vi "labpower.vi"() -> ()   [LabVIEW 2019]
panel:
  in  "Numeric":dbl
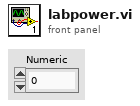
[diagram p1: front panel]
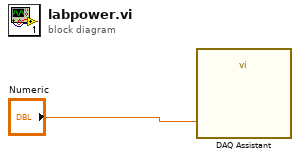
[diagram p0: block diagram]
diagram:
  n1 = call "DAQ Assistant"("data"="Numeric") -> ()  [unwired: 17 in, 2 out]
